vi "ProXR_IO_CONTROL.vi"(3 "error in (no error)":errorcluster {"code" format="%.0x"}, 4 "IO-port":T1(ring), 5 "VISA resource name":refnum<visa-resource-name>="COM1") -> (0 "error out":errorcluster, 1 "VISA resource name Out":refnum<visa-resource-name>, 2 "Receive_buffer":u8[](array[numeric]))   [LabVIEW 2014]
panel:
  out "Read Count":u32
  out "Write Count":u32
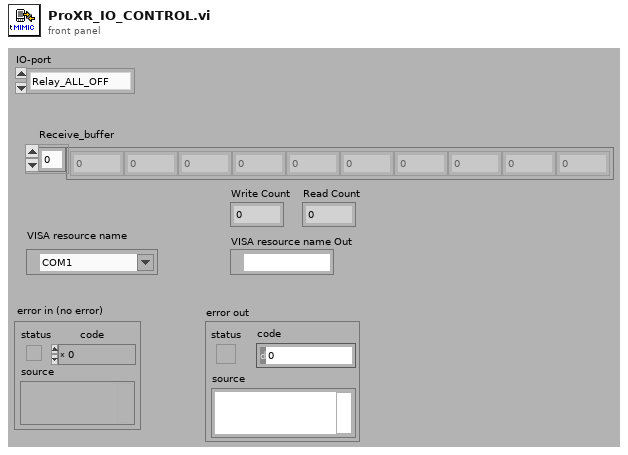
[diagram p1: front panel]
types:
  T1 = enum16{"Relay_ALL_OFF", "Relay_1_ON", "Relay_2_ON", "Relay_3_ON", "Relay_4_ON", "Relay_5_ON", "Relay_6_ON", "Relay_7_ON", "Relay_8_ON", "Relay_1_OFF", "Relay_2_OFF", "Relay_3_OFF", "Relay_4_OFF", "Relay_5_OFF", "Relay_6_OFF", "Relay_7_OFF", "Relay_8_OFF", "Read_AD_1", "Read_AD_2"}
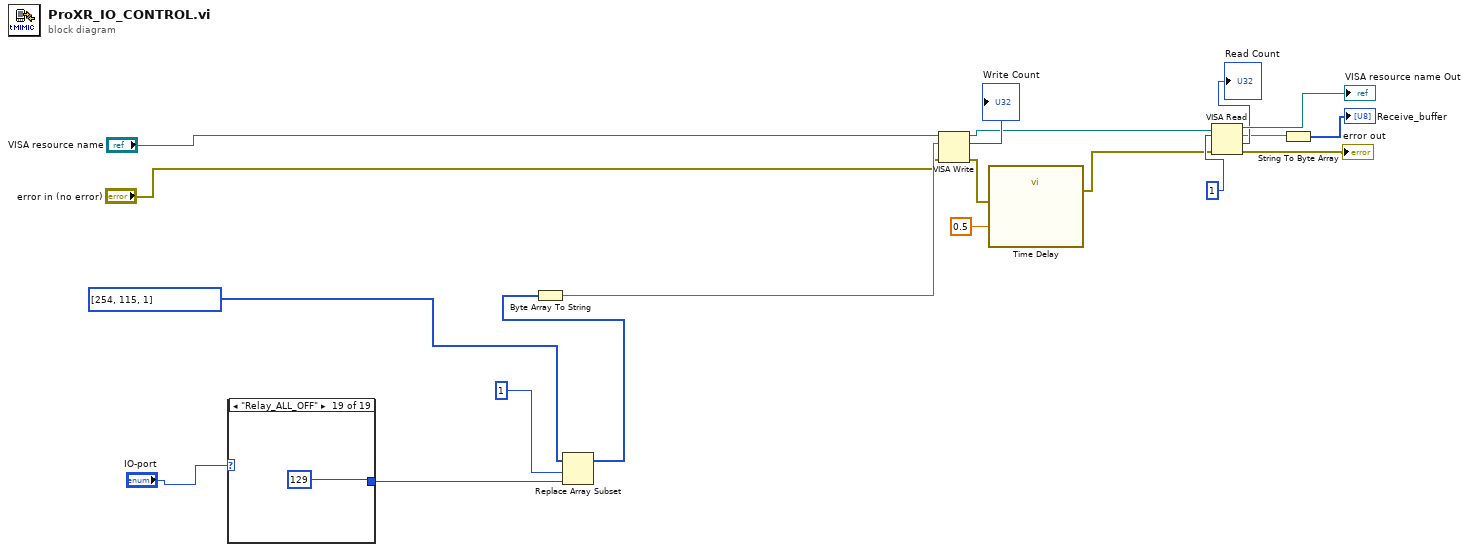
[diagram p0: block diagram]
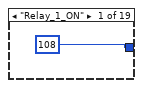
[diagram p2: hidden frame]
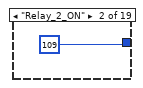
[diagram p3: hidden frame]
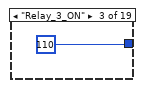
[diagram p4: hidden frame]
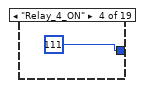
[diagram p5: hidden frame]
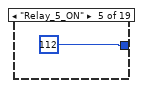
[diagram p6: hidden frame]
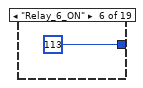
[diagram p7: hidden frame]
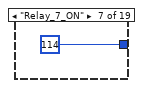
[diagram p8: hidden frame]
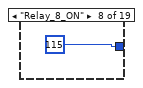
[diagram p9: hidden frame]
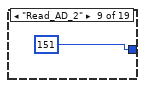
[diagram p10: hidden frame]
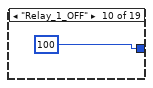
[diagram p11: hidden frame]
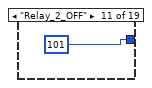
[diagram p12: hidden frame]
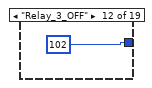
[diagram p13: hidden frame]
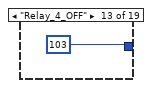
[diagram p14: hidden frame]
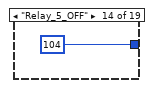
[diagram p15: hidden frame]
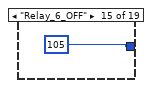
[diagram p16: hidden frame]
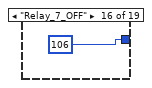
[diagram p17: hidden frame]
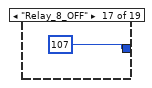
[diagram p18: hidden frame]
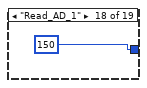
[diagram p19: hidden frame]
diagram:
  n1 = case shown="\"Relay_ALL_OFF\"" "IO-port" {
    tunnel: [108 ("index") 109 ("index") 110 ("index") 111 ("index") 112 ("index") 113 ("index") 114 ("index") 115 ("index") 151 ("index") 100 ("index") 101 ("index") 102 ("index") 103 ("index") 104 ("index") 105 ("index") 106 ("index") 107 ("index") 150 ("index") 129 ("index")] -> w1
    frame "Relay_1_ON" {
    }
    frame "Relay_2_ON" {
    }
    frame "Relay_3_ON" {
    }
    frame "Relay_4_ON" {
    }
    frame "Relay_5_ON" {
    }
    frame "Relay_6_ON" {
    }
    frame "Relay_7_ON" {
    }
    frame "Relay_8_ON" {
    }
    frame "Read_AD_2" {
    }
    frame "Relay_1_OFF" {
    }
    frame "Relay_2_OFF" {
    }
    frame "Relay_3_OFF" {
    }
    frame "Relay_4_OFF" {
    }
    frame "Relay_5_OFF" {
    }
    frame "Relay_6_OFF" {
    }
    frame "Relay_7_OFF" {
    }
    frame "Relay_8_OFF" {
    }
    frame "Read_AD_1" {
    }
    frame "Relay_ALL_OFF" {
    }
  }
  n2 = Replace Array Subset(array=u8[] [254, 115, 1] ("Command array"), new element=w1, index=1) -> (w3:u8[])
  n3 = Byte Array To String(unsigned byte array=w3) -> (string=w18:string)
  n4 = VISA Write(VISA resource name="VISA resource name", write buffer=w18, error in (no error)="error in (no error)") -> (VISA resource name out=w9:refnum<visa-resource-name>, return count=→"Write Count":u32, error out=w10:errorcluster)
  n5 = call "Time Delay"("error in (no error)"=w10, "Delay Time (s)"=0.5) -> ("error out"=w8:errorcluster)  [unwired: 9 in]
  n6 = VISA Read(VISA resource name=w9, byte count=u32 1, error in (no error)=w8) -> (VISA resource name out=→"VISA resource name Out":refnum<visa-resource-name>, read buffer=w13:string, return count=→"Read Count":u32, error out=→"error out":errorcluster)
  n7 = String To Byte Array(string=w13) -> (unsigned byte array=→"Receive_buffer":u8[])
